vi "ShowTime.vi"(9 "relative seconds":dbl, 10 "Value in":T1 {"Time Count" format="%.2g"}, 11 "Cluster in":refnum<vi>) -> (3 "Value out":T1 {"Time Count" format="%.2g"})   [LabVIEW 2016]
uses:
  Controls/Boiler Status Indicators.ctl
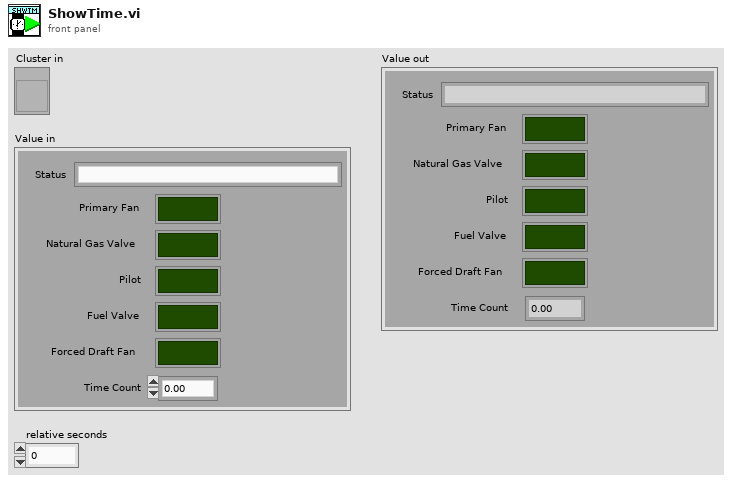
[diagram p1: front panel]
types:
  T1 = typedef "Boiler Status Indicators.ctl" = cluster{"Status":string, "Primary Fan":bool, "Natural Gas Valve":bool, "Pilot":bool, "Fuel Valve":bool, "Forced Draft Fan":bool, "Time Count":dbl}
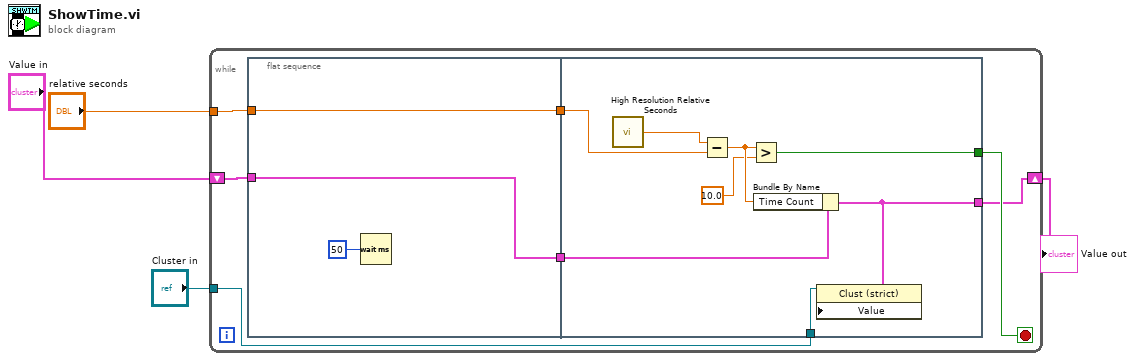
[diagram p0: block diagram]
diagram:
  n1 = while {
    tunnel: "relative seconds" -> [w10]
    shift-right: [w6] -> w4
    shift-left: "Value in" -> [w11]
    tunnel: "Cluster in" -> [w5]
    stop <- w7 stop-if-true
    n2 = flat-sequence {
      tunnel: w11 -> [w13]
      tunnel: w10 -> [w12]
      tunnel: [w13] -> w9
      tunnel: [w12] -> w8
      tunnel: w9 -> [w19]
      tunnel: w8 -> [w18]
      tunnel: [w17] -> w7
      tunnel: [w16] -> w6
      tunnel: w5 -> [w15]
      frame #0 {
        n3 = Wait (ms)(milliseconds to wait=u32 50) -> ()  [unwired: 1 out]
      }
      frame #1 {
        n4 = call <vilib>:"High Resolution Relative Seconds.vi"() -> ("relative seconds"=w20:dbl)
        n5 = Subtract(x=w20, y=w18) -> (x-y=w22:dbl)
        n6 = Greater?(x=w22, y=10.0) -> (0:w17:bool)
        n7 = Bundle By Name(cluster=w19, "Time Count"=w22) -> (w16:T1)
        n8 = property class="Clust (strict)"(reference=w15, "Value"=w16) -> ()  [unwired: 1 in, 2 out]
      }
    }
  }
  "Value out" <- w4
